vi "GEA2 Script Single.vi"(0 "GEA2 Reference In":refnum<k24>, 2 "Script line test name":string="Test", 5 "Script line":string, 7 "Default wait time (s)":dbl=0.25, 9 "Continue if failed?":bool=TRUE, 11 "Error In":errorcluster) -> (4 "GEA2 Reference Out":refnum<k24>, 6 "Pass/Fail?":bool, 8 "Report Text":string, 15 "Error Out":errorcluster)   [LabVIEW 2016]
doc: "Use this VI to execute a single line of a GEA2 script. Multiple lines can be executed."
uses:
  Q:/Common/DLLs/GEA3/GeaCommunication.dll
  DLLs/GEA3/GeaCommunication.dll
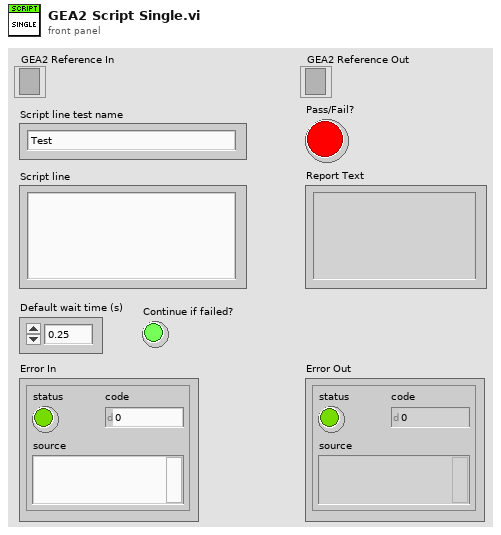
[diagram p1: front panel]
types:
  T1 = typedef "Script Output.ctl" = cluster{"Command Data":string[], "Command Type":T2[], "Test Name":string, "Wait Time (s)":dbl[], "Continue if failed?":bool[]}
  T2 = typedef "Command Type.ctl" = enum16{"WRITE", "READ", "ERDWRITE", "ERDREAD"}
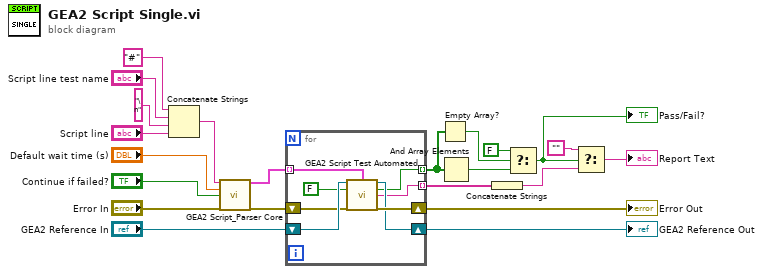
[diagram p0: block diagram]
diagram:
  n1 = Concatenate Strings("#" ("string"), "Script line test name", "\n" ("string"), "Script line") -> (w22:string)
  n2 = call "GEA2 Script_Parser Core.vi"("Script In"=w22, "Default wait time (s)"="Default wait time (s)", "Default continue if failed?"="Continue if failed?", "Error In"="Error In") -> ("Script Output"=w19:T1[], "Error Out"=w17:errorcluster)  [unwired: 10 in]
  n3 = for {
    tunnel: w19 -> [w28] mode=indexing
    shift-right: [w27] -> w18
    shift-left: w17 -> [w26]
    shift-right: [w25] -> w13
    shift-left: "GEA2 Reference In" -> [w30]
    tunnel: [w24] -> w12 mode=indexing
    tunnel: [w23] -> w9 mode=indexing
    n4 = call "GEA2 Script Test Automated.vi"("GEA2 Reference In"=w30, "Test Case"=w28, "Standalone"=FALSE, "Error In"=w26) -> ("GEA2 Reference Out"=w25:refnum<k24>, "Pass/Fail?"=w24:bool, "Report Text"=w23:string, "Error Out"=w27:errorcluster)  [unwired: 8 in]
  }
  "Error Out" <- w18
  "GEA2 Reference Out" <- w13
  n5 = Empty Array?(array=w12) -> (empty?=w11:bool)
  n6 = And Array Elements(Boolean array=w12) -> (logical AND=w10:bool)
  n7 = Concatenate Strings(w9) -> (w6:string)
  n8 = Select(t=FALSE, s=w11, f=w10) -> (s? t:f=w7:bool)
  "Pass/Fail?" <- w7
  n9 = Select(t="", s=w7, f=w6) -> (s? t:f=→"Report Text":string)
